vi "SW_Load_settings_to_main_tab.vi"(0 "Refnum in":T4=refnum, 2 "User Name":string="Admin", 3 "error in (no error)":errorcluster) -> (4 "VISA resource name":string, 6 "Refnum out":T4, 7 "IO parameters cluster":T2, 8 "Settings cluster out":T1, 9 "Stimulus presets array":T3(array[cluster])=[{"Event type"=0, "Dur., s"=0.0, "Stim., s"=0.0, "Set/Clear"=FALSE, "TTL out N"=1, "Stim. has been set"=FALSE}, {"Event type"=0, "Dur., s"=0.0, "Stim., s"=0.0, "Set/Clear"=FALSE, "TTL out N"=1, "Stim. has been set"=FALSE}, {"Event type"=0, "Dur., s"=0.0, "Stim., s"=0.0, "Set/Clear"=FALSE, "TTL out N"=1, "Stim. has been set"=FALSE}, {"Event type"=0, "Dur., s"=0.0, "Stim., s"=0.0, "Set/Clear"=FALSE, "TTL out N"=1, "Stim. has been set"=FALSE}, {"Event type"=0, "Dur., s"=0.0, "Stim., s"=0.0, "Set/Clear"=FALSE, "TTL out N"=1, "Stim. has been set"=FALSE}, {"Event type"=0, "Dur., s"=0.0, "Stim., s"=0.0, "Set/Clear"=FALSE, "TTL out N"=1, "Stim. has been set"=FALSE}, {"Event type"=0, "Dur., s"=0.0, "Stim., s"=0.0, "Set/Clear"=FALSE, "TTL out N"=1, "Stim. has been set"=FALSE}, {"Event type"=0, "Dur., s"=0.0, "Stim., s"=0.0, "Set/Clear"=FALSE, "TTL out N"=1, "Stim. has been set"=FALSE}, {"Event type"=0, "Dur., s"=0.0, "Stim., s"=0.0, "Set/Clear"=FALSE, "TTL out N"=1, "Stim. has been set"=FALSE}, {"Event type"=0, "Dur., s"=0.0, "Stim., s"=0.0, "Set/Clear"=FALSE, "TTL out N"=1, "Stim. has been set"=FALSE}, {"Event type"=0, "Dur., s"=0.0, "Stim., s"=0.0, "Set/Clear"=FALSE, "TTL out N"=1, "Stim. has been set"=FALSE}, {"Event type"=0, "Dur., s"=0.0, "Stim., s"=0.0, "Set/Clear"=FALSE, "TTL out N"=1, "Stim. has been set"=FALSE}, {"Event type"=0, "Dur., s"=0.0, "Stim., s"=0.0, "Set/Clear"=FALSE, "TTL out N"=1, "Stim. has been set"=FALSE}, {"Event type"=0, "Dur., s"=0.0, "Stim., s"=0.0, "Set/Clear"=FALSE, "TTL out N"=1, "Stim. has been set"=FALSE}] {"Event type" items=["Stay for N seconds"]; "TTL out N" items=["1"=1, "2"=2, "1+2"=3]}, 10 "error out":errorcluster={"status"=TRUE, "code"=1, "source"="Dequeue Element in NI_LVConfig.lvlib:Read Value Without Comment.vi->NI_LVConfig.lvlib:Read Key (I32).vi->SW_Load_settings_to_main_tab.vi"})   [LabVIEW 2018, in "Tracker.lvlib"]
uses:
  Tracker.lvlib
  <vilib>/Utility/config.llb/Config Data RefNum.ctl
  <vilib>/Utility/config.llb/NI_LVConfig.lvlib
panel:
  out "Data filtering choice":u16=180
  out "\"Stop at\" enabled":bool
  out "Name prefix":string
  out "Stop at":dbl
  out "Offset H.":dbl
  out "Twisted neck":bool
  out "Vertical offset":dbl
  out "Bridge swap?":bool
  out "Cage diameter, mm":i32=180
  out "Border segments starting angle":i32
  out "Midfield segments starting angle":i32
  out "Midfield segments outer radius, mm":i32=60
  out "Center segment outer radius, mm":i32=30
  out "Amount of border segments":i32=8
  out "Amount of midfield segments":i32=4
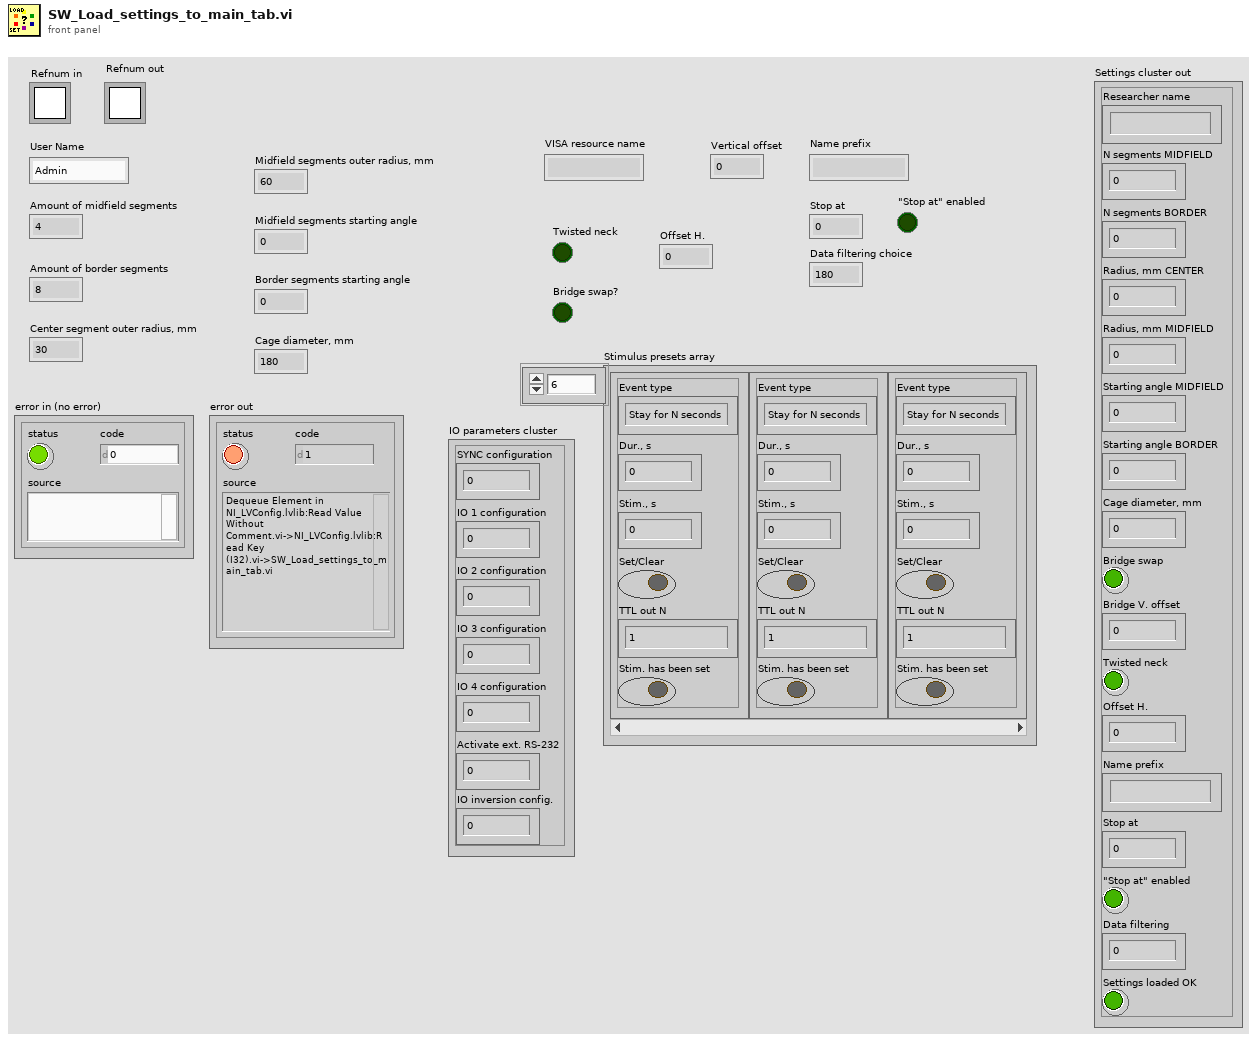
[diagram p1: front panel]
types:
  T1 = cluster{"Researcher name":string, "N segments MIDFIELD":u8, "N segments BORDER":u8, "Radius, mm CENTER":u16, "Radius, mm MIDFIELD":u16, "Starting angle MIDFIELD":i16, "Starting angle BORDER":i16, "Cage diameter, mm":u16, "Bridge swap":bool, "Bridge V. offset":sgl, "Twisted neck":bool, "Offset H.":sgl, "Name prefix":string, "Stop at":dbl, "\"Stop at\" enabled":bool, "Data filtering":u16, "Settings loaded OK":bool}
  T2 = cluster{"SYNC configuration":u16, "IO 1 configuration":u16, "IO 2 configuration":u16, "IO 3 configuration":u16, "IO 4 configuration":u16, "Activate ext. RS-232":u16, "IO inversion config.":u16}
  T3 = cluster{"Event type":u16, "Dur., s":sgl, "Stim., s":sgl, "Set/Clear":bool, "TTL out N":u16, "Stim. has been set":bool}[]
  T4 = typedef "NI_LVConfig.lvlib/Config Data RefNum.ctl" = refnum<k1>
  T5 = cluster{"array[0]":u16, "array[1]":u16, "array[2]":u16, "array[3]":u16, "array[4]":u16, "array[5]":u16, "array[6]":u16, "array[7]":u16, "array[8]":u16}
  T6 = cluster{"Event type":u16, "Time, s":sgl, "Stimulus, s":sgl, "Set/Clear":bool, "TTL out":u16, "Stim. has been set":bool}
  T7 = cluster{"Event type":u16, "Cond., s":sgl, "Stim., s":sgl, "Set/Clear":bool, "TTL out N":u16, "Stim. has been set":bool}
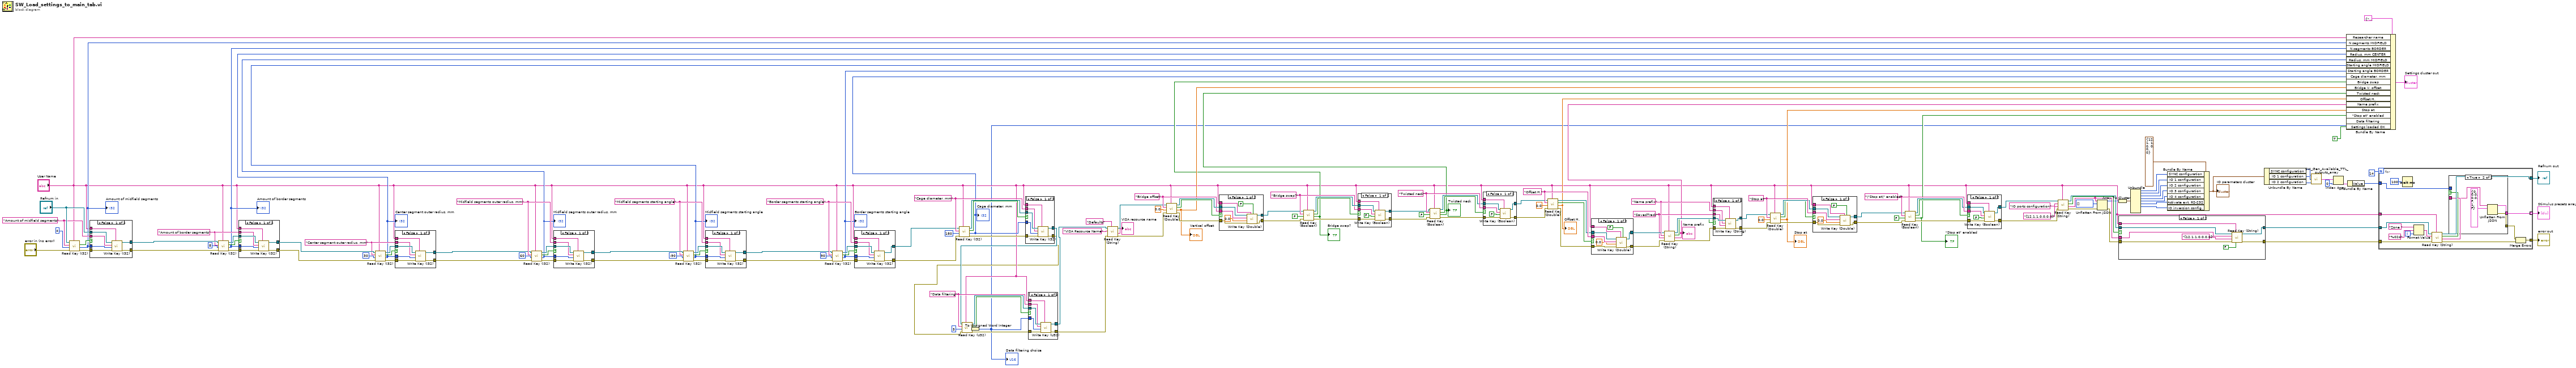
[diagram p0: block diagram]
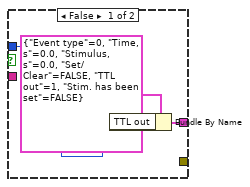
[diagram p8: hidden frame]
diagram:
  w12 = "Data filtering" ("key")
  w37 = "\"Stop at\" enabled"
  w46 = "Stop at" ("key")
  w41 = "SavedTrack" ("default value")
  w49 = "Name prefix"
  w59 = "Offset H." ("key")
  w65 = "Twisted neck"
  w101 = "Bridge offset" ("key")
  w109 = "Bridge swap?"
  w118 = "Cage diameter, mm" ("key")
  w129 = "Border segments starting angle" ("key")
  w130 = "Midfield segments starting angle" ("key")
  w142 = "Midfield segments outer radius, mm" ("key")
  w145 = "Center segment outer radius, mm" ("key")
  w151 = "Amount of border segments" ("key")
  w160 = "Amount of midfield segments" ("key")
  n1 = call <vilib>:"Read Key (I32).vi"("section"="User Name", "error in (no error)"="error in (no error)", "default value"=4, "key"=w160, "refnum"="Refnum in") -> ("error out"=w158:errorcluster, "value"=w28:i32, "found?"=w162:bool)  [unwired: 3 in, 1 out]
  "Amount of midfield segments" <- w28
  n2 = case shown="False" w162 {
    tunnel: "User Name" -> [w169 _]
    tunnel: "Refnum in" -> [w170 w172]
    tunnel: w160 -> [w168 _]
    tunnel: w28 -> [w167 _]
    tunnel: w158 -> [w166 w171]
    tunnel: [w165 w171] -> w155
    tunnel: [w164 w172] -> w157
    frame False {
      n3 = call <vilib>:"Write Key (I32).vi"("section"=w169, "error in (no error)"=w166, "value"=w167, "key"=w168, "refnum"=w170) -> ("error out"=w165:errorcluster, "refnum out"=w164:T4)  [unwired: 4 in, 1 out]
    }
    frame True {
    }
  }
  n4 = call <vilib>:"Read Key (I32).vi"("section"="User Name", "error in (no error)"=w155, "default value"=8, "key"=w151, "refnum"=w157) -> ("error out"=w152:errorcluster, "value"=w27:i32, "found?"=w153:bool, "refnum out"=w154:T4)  [unwired: 3 in]
  "Amount of border segments" <- w27
  n5 = case shown="False" w153 {
    tunnel: "User Name" -> [w178 _]
    tunnel: w154 -> [w179 w181]
    tunnel: w151 -> [w177 _]
    tunnel: w27 -> [w176 _]
    tunnel: w152 -> [w175 w180]
    tunnel: [w174 w180] -> w147
    tunnel: [w173 w181] -> w146
    frame False {
      n6 = call <vilib>:"Write Key (I32).vi"("section"=w178, "error in (no error)"=w175, "value"=w176, "key"=w177, "refnum"=w179) -> ("error out"=w174:errorcluster, "refnum out"=w173:T4)  [unwired: 4 in, 1 out]
    }
    frame True {
    }
  }
  n7 = call <vilib>:"Read Key (I32).vi"("section"="User Name", "error in (no error)"=w147, "default value"=30, "key"=w145, "refnum"=w146) -> ("error out"=w150:errorcluster, "value"=w26:i32, "found?"=w149:bool, "refnum out"=w148:T4)  [unwired: 3 in]
  "Center segment outer radius, mm" <- w26
  n8 = case shown="False" w149 {
    tunnel: "User Name" -> [w187 _]
    tunnel: w148 -> [w188 w190]
    tunnel: w145 -> [w186 _]
    tunnel: w26 -> [w185 _]
    tunnel: w150 -> [w184 w189]
    tunnel: [w183 w189] -> w138
    tunnel: [w182 w190] -> w137
    frame False {
      n9 = call <vilib>:"Write Key (I32).vi"("section"=w187, "error in (no error)"=w184, "value"=w185, "key"=w186, "refnum"=w188) -> ("error out"=w183:errorcluster, "refnum out"=w182:T4)  [unwired: 4 in, 1 out]
    }
    frame True {
    }
  }
  n10 = call <vilib>:"Read Key (I32).vi"("section"="User Name", "error in (no error)"=w138, "default value"=60, "key"=w142, "refnum"=w137) -> ("error out"=w139:errorcluster, "value"=w25:i32, "found?"=w140:bool, "refnum out"=w141:T4)  [unwired: 3 in]
  "Midfield segments outer radius, mm" <- w25
  n11 = case shown="False" w140 {
    tunnel: "User Name" -> [w196 _]
    tunnel: w141 -> [w197 w199]
    tunnel: w142 -> [w195 _]
    tunnel: w25 -> [w194 _]
    tunnel: w139 -> [w193 w198]
    tunnel: [w192 w198] -> w132
    tunnel: [w191 w199] -> w131
    frame False {
      n12 = call <vilib>:"Write Key (I32).vi"("section"=w196, "error in (no error)"=w193, "value"=w194, "key"=w195, "refnum"=w197) -> ("error out"=w192:errorcluster, "refnum out"=w191:T4)  [unwired: 4 in, 1 out]
    }
    frame True {
    }
  }
  n13 = call <vilib>:"Read Key (I32).vi"("section"="User Name", "error in (no error)"=w132, "default value"=-90, "key"=w130, "refnum"=w131) -> ("error out"=w136:errorcluster, "value"=w24:i32, "found?"=w135:bool, "refnum out"=w134:T4)  [unwired: 3 in]
  "Midfield segments starting angle" <- w24
  n14 = case shown="False" w135 {
    tunnel: "User Name" -> [w205 _]
    tunnel: w134 -> [w206 w208]
    tunnel: w130 -> [w204 _]
    tunnel: w24 -> [w203 _]
    tunnel: w136 -> [w202 w207]
    tunnel: [w201 w207] -> w123
    tunnel: [w200 w208] -> w124
    frame False {
      n15 = call <vilib>:"Write Key (I32).vi"("section"=w205, "error in (no error)"=w202, "value"=w203, "key"=w204, "refnum"=w206) -> ("error out"=w201:errorcluster, "refnum out"=w200:T4)  [unwired: 4 in, 1 out]
    }
    frame True {
    }
  }
  n16 = call <vilib>:"Read Key (I32).vi"("section"="User Name", "error in (no error)"=w123, "default value"=90, "key"=w129, "refnum"=w124) -> ("error out"=w125:errorcluster, "value"=w23:i32, "found?"=w126:bool, "refnum out"=w127:T4)  [unwired: 3 in]
  "Border segments starting angle" <- w23
  n17 = case shown="False" w126 {
    tunnel: "User Name" -> [w214 _]
    tunnel: w127 -> [w215 w217]
    tunnel: w129 -> [w213 _]
    tunnel: w23 -> [w212 _]
    tunnel: w125 -> [w211 w216]
    tunnel: [w210 w216] -> w116
    tunnel: [w209 w217] -> w117
    frame False {
      n18 = call <vilib>:"Write Key (I32).vi"("section"=w214, "error in (no error)"=w211, "value"=w212, "key"=w213, "refnum"=w215) -> ("error out"=w210:errorcluster, "refnum out"=w209:T4)  [unwired: 4 in, 1 out]
    }
    frame True {
    }
  }
  n19 = call <vilib>:"Read Key (I32).vi"("section"="User Name", "error in (no error)"=w116, "default value"=180, "key"=w118, "refnum"=w117) -> ("error out"=w122:errorcluster, "value"=w22:i32, "found?"=w121:bool, "refnum out"=w120:T4)  [unwired: 3 in]
  "Cage diameter, mm" <- w22
  n20 = case shown="False" w121 {
    tunnel: "User Name" -> [w223 _]
    tunnel: w120 -> [w224 w226]
    tunnel: w118 -> [w222 _]
    tunnel: w22 -> [w221 _]
    tunnel: w122 -> [w220 w225]
    tunnel: [w219 w225] -> w4
    tunnel: [w218 w226] -> w6
    frame False {
      n21 = call <vilib>:"Write Key (I32).vi"("section"=w223, "error in (no error)"=w220, "value"=w221, "key"=w222, "refnum"=w224) -> ("error out"=w219:errorcluster, "refnum out"=w218:T4)  [unwired: 4 in, 1 out]
    }
    frame True {
    }
  }
  n22 = call <vilib>:"Read Key (U32).vi"("section"="User Name", "error in (no error)"=w4, "default value"=5, "key"=w12, "refnum"=w6) -> ("error out"=w8:errorcluster, "value"=w13:u32, "found?"=w9:bool, "refnum out"=w10:T4)  [unwired: 3 in]
  n23 = To Unsigned Word Integer(number=w13) -> (unsigned 16bit integer=w2:u16)
  "Data filtering choice" <- w2
  n24 = case shown="False" w9 {
    tunnel: "User Name" -> [w232 _]
    tunnel: w10 -> [w233 w235]
    tunnel: w12 -> [w231 _]
    tunnel: w2 -> [w230 _]
    tunnel: w8 -> [w229 w234]
    tunnel: [w228 w234] -> w3
    tunnel: [w227 w235] -> w5
    frame False {
      n25 = call <vilib>:"Write Key (U32).vi"("section"=w232, "error in (no error)"=w229, "value"=w230, "key"=w231, "refnum"=w233) -> ("error out"=w228:errorcluster, "refnum out"=w227:T4)  [unwired: 4 in, 1 out]
    }
    frame True {
    }
  }
  n26 = call <vilib>:"Read Key (String).vi"("section"="Defaults", "error in (no error)"=w3, "key"="VISA Resource Name", "refnum"=w5) -> ("error out"=w83:errorcluster, "value"=→"VISA resource name":string, "refnum out"=w82:T4)  [unwired: 4 in, 1 out]
  n27 = call <vilib>:"Read Key (Double).vi"("section"="User Name", "error in (no error)"=w83, "default value"=0.0, "key"=w101, "refnum"=w82) -> ("error out"=w105:errorcluster, "value"=w21:dbl, "found?"=w103:bool, "refnum out"=w102:T4)  [unwired: 3 in]
  "Vertical offset" <- w21
  n28 = case shown="False" w103 {
    tunnel: [w241 w244] -> w106
    tunnel: [w242 w245] -> w107
    tunnel: w105 -> [w243 w245]
    tunnel: "User Name" -> [w240 _]
    tunnel: w101 -> [w239 _]
    tunnel: w102 -> [w237 w244]
    frame False {
      n29 = call <vilib>:"Write Key (Double).vi"("use system decimal point (T)"=FALSE ("value"), "section"=w240, "error in (no error)"=w243, "value"=0.0, "key"=w239, "refnum"=w237) -> ("error out"=w242:errorcluster, "refnum out"=w241:T4)  [unwired: 3 in, 1 out]
    }
    frame True {
    }
  }
  n30 = call <vilib>:"Read Key (Boolean).vi"("section"="User Name", "error in (no error)"=w107, "default value"=FALSE, "key"=w109, "refnum"=w106) -> ("error out"=w111:errorcluster, "value"=w20:bool, "found?"=w110:bool, "refnum out"=w112:T4)  [unwired: 3 in]
  "Bridge swap?" <- w20
  n31 = case shown="False" w110 {
    tunnel: w112 -> [w250 w254]
    tunnel: [w249 w254] -> w61
    tunnel: [w251 w253] -> w60
    tunnel: w111 -> [w252 w253]
    tunnel: "User Name" -> [w248 _]
    tunnel: w109 -> [w247 _]
    frame False {
      n32 = call <vilib>:"Write Key (Boolean).vi"("section"=w248, "error in (no error)"=w252, "value"=FALSE, "key"=w247, "refnum"=w250) -> ("error out"=w251:errorcluster, "refnum out"=w249:T4)  [unwired: 4 in, 1 out]
    }
    frame True {
    }
  }
  n33 = call <vilib>:"Read Key (Boolean).vi"("section"="User Name", "error in (no error)"=w60, "default value"=FALSE, "key"=w65, "refnum"=w61) -> ("error out"=w63:errorcluster, "value"=w19:bool, "found?"=w64:bool, "refnum out"=w62:T4)  [unwired: 3 in]
  "Twisted neck" <- w19
  n34 = case shown="False" w64 {
    tunnel: w62 -> [w259 w263]
    tunnel: [w258 w263] -> w54
    tunnel: [w260 w262] -> w53
    tunnel: w63 -> [w261 w262]
    tunnel: "User Name" -> [w257 _]
    tunnel: w65 -> [w256 _]
    frame False {
      n35 = call <vilib>:"Write Key (Boolean).vi"("section"=w257, "error in (no error)"=w261, "value"=FALSE, "key"=w256, "refnum"=w259) -> ("error out"=w260:errorcluster, "refnum out"=w258:T4)  [unwired: 4 in, 1 out]
    }
    frame True {
    }
  }
  n36 = call <vilib>:"Read Key (Double).vi"("section"="User Name", "error in (no error)"=w53, "default value"=0.0, "key"=w59, "refnum"=w54) -> ("error out"=w55:errorcluster, "value"=w18:dbl, "found?"=w57:bool, "refnum out"=w58:T4)  [unwired: 3 in]
  "Offset H." <- w18
  n37 = case shown="False" w57 {
    tunnel: [w269 w272] -> w47
    tunnel: [w270 w273] -> w48
    tunnel: w55 -> [w271 w273]
    tunnel: "User Name" -> [w268 _]
    tunnel: w59 -> [w267 _]
    tunnel: w58 -> [w265 w272]
    frame False {
      n38 = call <vilib>:"Write Key (Double).vi"("use system decimal point (T)"=FALSE ("value"), "section"=w268, "error in (no error)"=w271, "value"=0.0, "key"=w267, "refnum"=w265) -> ("error out"=w270:errorcluster, "refnum out"=w269:T4)  [unwired: 3 in, 1 out]
    }
    frame True {
    }
  }
  n39 = call <vilib>:"Read Key (String).vi"("section"="User Name", "error in (no error)"=w48, "default value"=w41, "key"=w49, "refnum"=w47) -> ("error out"=w51:errorcluster, "value"=w17:string, "found?"=w50:bool, "refnum out"=w52:T4)  [unwired: 3 in]
  "Name prefix" <- w17
  n40 = case shown="False" w50 {
    tunnel: w52 -> [w278 w282]
    tunnel: [w277 w282] -> w40
    tunnel: [w279 w281] -> w39
    tunnel: w51 -> [w280 w281]
    tunnel: "User Name" -> [w276 _]
    tunnel: w49 -> [w275 _]
    tunnel: w41 -> [w274 _]
    frame False {
      n41 = call <vilib>:"Write Key (String).vi"("section"=w276, "error in (no error)"=w280, "value"=w274, "key"=w275, "refnum"=w278) -> ("error out"=w279:errorcluster, "refnum out"=w277:T4)  [unwired: 4 in, 1 out]
    }
    frame True {
    }
  }
  n42 = call <vilib>:"Read Key (Double).vi"("section"="User Name", "error in (no error)"=w39, "default value"=0.0, "key"=w46, "refnum"=w40) -> ("error out"=w42:errorcluster, "value"=w16:dbl, "found?"=w44:bool, "refnum out"=w45:T4)  [unwired: 3 in]
  "Stop at" <- w16
  n43 = case shown="False" w44 {
    tunnel: [w288 w291] -> w33
    tunnel: [w289 w292] -> w32
    tunnel: w42 -> [w290 w292]
    tunnel: "User Name" -> [w287 _]
    tunnel: w46 -> [w286 _]
    tunnel: w45 -> [w284 w291]
    frame False {
      n44 = call <vilib>:"Write Key (Double).vi"("use system decimal point (T)"=FALSE ("value"), "section"=w287, "error in (no error)"=w290, "value"=0.0, "key"=w286, "refnum"=w284) -> ("error out"=w289:errorcluster, "refnum out"=w288:T4)  [unwired: 3 in, 1 out]
    }
    frame True {
    }
  }
  n45 = call <vilib>:"Read Key (Boolean).vi"("section"="User Name", "error in (no error)"=w32, "default value"=FALSE, "key"=w37, "refnum"=w33) -> ("error out"=w35:errorcluster, "value"=w15:bool, "found?"=w36:bool, "refnum out"=w34:T4)  [unwired: 3 in]
  "\"Stop at\" enabled" <- w15
  n46 = case shown="False" w36 {
    tunnel: w34 -> [w297 w301]
    tunnel: [w296 w301] -> w31
    tunnel: [w298 w300] -> w30
    tunnel: w35 -> [w299 w300]
    tunnel: "User Name" -> [w295 _]
    tunnel: w37 -> [w294 _]
    frame False {
      n47 = call <vilib>:"Write Key (Boolean).vi"("section"=w295, "error in (no error)"=w299, "value"=FALSE, "key"=w294, "refnum"=w297) -> ("error out"=w298:errorcluster, "refnum out"=w296:T4)  [unwired: 4 in, 1 out]
    }
    frame True {
    }
  }
  n48 = call <vilib>:"Read Key (String).vi"("section"="User Name", "error in (no error)"=w30, "default value"="[12,1,1,0,0,0,0]" ("IO parameters string"), "key"="IO ports configuration", "refnum"=w31) -> ("error out"=w95:errorcluster, "value"=w96:string, "found?"=w99:bool, "refnum out"=w98:T4)  [unwired: 3 in]
  n49 = Unflatten From JSON(JSON string=w96, type and defaults=u16[] [] ("array"), error in (no error)=w95) -> (value=w93:u16[], error out=w94:errorcluster)  [unwired: 4 in]
  n50 = Array To Cluster(array=w93) -> (cluster=w91:T5)
  n51 = case shown="False" w99 {
    tunnel: w98 -> [w307 w311]
    tunnel: [w306 w311] -> w78
    tunnel: [w308 w310] -> w80
    tunnel: w94 -> [w309 w310]
    tunnel: "User Name" -> [w305 _]
    tunnel: w96 -> [w304 _]
    frame False {
      n52 = call <vilib>:"Read Key (String).vi"("read raw string? (F)"=FALSE ("value"), "section"=w305, "error in (no error)"=w309, "default value"="[12,1,1,0,0,0,0]" ("IO parameters string"), "key"=w304, "refnum"=w307) -> ("error out"=w308:errorcluster, "refnum out"=w306:T4)  [unwired: 2 in, 2 out]
    }
    frame True {
    }
  }
  n53 = Unbundle(w91) -> ("array[0]"=w90:u16, "array[1]"=w89:u16, "array[2]"=w88:u16, "array[3]"=w87:u16, "array[4]"=w86:u16, "array[5]"=w85:u16, "array[6]"=w67:u16)  [unwired: 2 out]
  n54 = Bundle By Name(cluster=T2 {"SYNC configuration"=12, "IO 1 configuration"=1, "IO 2 configuration"=1, "IO 3 configuration"=0, "IO 4 configuration"=0, "Activate ext. RS-232"=0, "IO inversion config."=0} ("Sync parameters cluster output"), "SYNC configuration"=w90, "IO 1 configuration"=w89, "IO 2 configuration"=w88, "IO 3 configuration"=w87, "IO 4 configuration"=w86, "Activate ext. RS-232"=w85, "IO inversion config."=w67) -> (w74:T2)
  "IO parameters cluster" <- w74
  n55 = Unbundle By Name(w74) -> ("SYNC configuration"=w75:u16, "IO 1 configuration"=w69:u16, "IO 2 configuration"=w68:u16)
  n56 = call "SW_Gen_Available_TTL_outputs_array.vi"("IO 2 configuration"=w68, "IO 1 configuration"=w69, "SYNC configuration"=w75) -> ("Available TTL outputs array"=w71:cluster{"String":string, "Value":i32}[])
  n57 = Index Array(array=w71, index=0) -> (element=w72:cluster{"String":string, "Value":i32})
  n58 = Bundle By Name(cluster=T1 {"Researcher name"="Researcher", "N segments MIDFIELD"=4, "N segments BORDER"=0, "Radius, mm CENTER"=30, "Radius, mm MIDFIELD"=75, "Starting angle MIDFIELD"=0, "Starting angle BORDER"=0, "Cage diameter, mm"=180, "Bridge swap"=FALSE, "Bridge V. offset"=0.0, "Twisted neck"=FALSE, "Offset H."=0.0, "Name prefix"="SavedTrack", "Stop at"=0.0, "\"Stop at\" enabled"=FALSE, "Data filtering"=5, "Settings loaded OK"=FALSE} ("Settings cluster out"), "Researcher name"="User Name", "N segments MIDFIELD"=w28, "N segments BORDER"=w27, "Radius, mm CENTER"=w26, "Radius, mm MIDFIELD"=w25, "Starting angle MIDFIELD"=w24, "Starting angle BORDER"=w23, "Cage diameter, mm"=w22, "Bridge swap"=w20, "Bridge V. offset"=w21, "Twisted neck"=w19, "Offset H."=w18, "Name prefix"=w17, "Stop at"=w16, "\"Stop at\" enabled"=w15, "Data filtering"=w2, "Settings loaded OK"=TRUE) -> (→"Settings cluster out":T1)
  n59 = Unbundle By Name(w72) -> ("Value"=w70:i32)
  n60 = for {
    N: 14 -> [_]
    tunnel: w78 -> [w325]
    tunnel: [w324] -> w77
    tunnel: "User Name" -> [w323]
    tunnel: w80 -> [w321]
    tunnel: [w315] -> w79
    tunnel: [w318] -> w76 mode=indexing
    tunnel: w70 -> [w312]
    i -> [w316]
    n61 = Wait (ms)(milliseconds to wait=u32 100) -> ()  [unwired: 1 out]
    n62 = Format Value(string ("")="Zone ", format string="%02d", value (0)=w316) -> (output string=w322:string)
    n63 = call <vilib>:"Read Key (String).vi"("section"=w323, "error in (no error)"=w321, "key"=w322, "refnum"=w325) -> ("error out"=w320:errorcluster, "value"=w319:string, "found?"=w317:bool, "refnum out"=w324:T4)  [unwired: 4 in]
    n64 = case shown="True" w317 {
      tunnel: w319 -> [_ w334]
      tunnel: [w329 w333] -> w318
      tunnel: [_ w332] -> w314
      tunnel: w312 -> [w328 _]
      frame False {
        n65 = Bundle By Name(cluster=T6 {"Event type"=0, "Time, s"=0.0, "Stimulus, s"=0.0, "Set/Clear"=FALSE, "TTL out"=1, "Stim. has been set"=FALSE} ("Cluster of the stimuls settings"), "TTL out"=w328) -> (w329:T6)
      }
      frame True {
        n66 = Unflatten From JSON(JSON string=w334, type and defaults=T7 {"Event type"=0, "Cond., s"=0.0, "Stim., s"=0.0, "Set/Clear"=FALSE, "TTL out N"=1, "Stim. has been set"=FALSE} ("Cluster of the stimuls settings")) -> (value=w333:T7, error out=w332:errorcluster)  [unwired: 5 in]
      }
    }
    n67 = Merge Errors(w314, w320) -> (w315:errorcluster)
  }
  "error out" <- w79
  "Refnum out" <- w77
  "Stimulus presets array" <- w76
